vi "TrajectoryUtil_MakeWeightedWayPoint_ENG.vi"(8 "Weight":dbl, 9 "Travel Angle DEG":dbl, 10 "Y_FT":dbl, 11 "X_FT":dbl) -> (3 "WEIGHTED_WAYPOINT":T1={"TRANSLATION"={"X"=0.0, "Y"=0.0}, "ROTATION"={"VALUE"=0.0, "COS"=1.0, "SIN"=0.0}, "SCALAR"=0.0} {"SCALAR" format="%14.3f"; "ROTATION"."SIN" format="%13.4f"; "ROTATION"."COS" format="%13.4f"; "ROTATION"."VALUE" format="%13.4f"; "TRANSLATION"."Y" format="%14.3f"; "TRANSLATION"."X" format="%14.3f"})   [LabVIEW 2019, in "Trajectory_Library.lvlib"]
doc: "Creates a waypoint data structure from individual inputs. \n\nInputs are all ENG units (Feet, Degrees) Output waypoint is SI units."
uses:
  Trajectory_Library.lvlib
  TRANSLATION2D.ctl
  ROTATION2D.ctl
  WEIGHTED_WAYPOINT.ctl
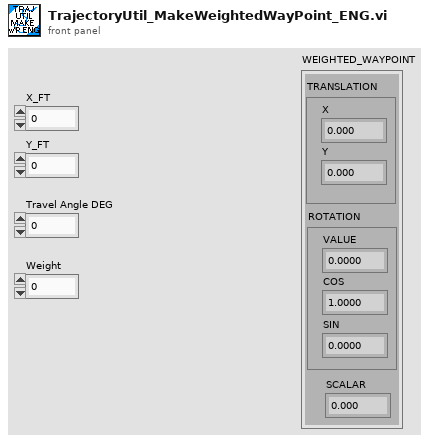
[diagram p1: front panel]
types:
  T1 = typedef "Trajectory_Library.lvlib/WEIGHTED_WAYPOINT.ctl" = cluster{"TRANSLATION":T2, "ROTATION":T3, "SCALAR":dbl}
  T2 = typedef "Trajectory_Library.lvlib/TRANSLATION2D.ctl" = cluster{"X":dbl, "Y":dbl}
  T3 = typedef "Trajectory_Library.lvlib/ROTATION2D.ctl" = cluster{"VALUE":dbl, "COS":dbl, "SIN":dbl}
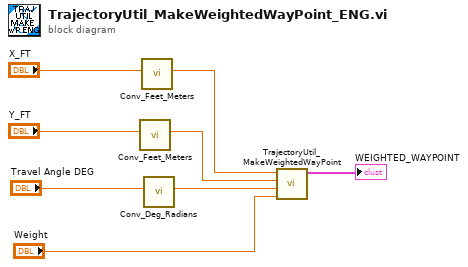
[diagram p0: block diagram]
diagram:
  n1 = call "Conv_Feet_Meters.vi"("Feet"="Y_FT") -> ("Meters"=w5:dbl)  [unwired: 10 in]
  n2 = call "Conv_Feet_Meters.vi"("Feet"="X_FT") -> ("Meters"=w4:dbl)  [unwired: 10 in]
  n3 = call "Conv_Deg_Radians.vi"("Degress"="Travel Angle DEG") -> ("Radians"=w6:dbl)  [unwired: 10 in]
  n4 = call "TrajectoryUtil_MakeWeightedWayPoint.vi"("Weight"="Weight", "Travel Angle Radians"=w6, "Y_M"=w5, "X_M"=w4) -> ("WEIGHTED_WAYPOINT"=→"WEIGHTED_WAYPOINT":T1)  [unwired: 7 in]
